vi "Read Payload.vi"(8 "error in (no error)":errorcluster, 11 "RDS Message in":refnum<class "RDS Message.lvclass">) -> (0 "error out":errorcluster, 2 "Payload Out":refnum<class "RDS Payload.lvclass">, 3 "RDS Message out":refnum<class "RDS Message.lvclass">)   [LabVIEW 2015]
uses:
  RDS Message.lvclass
  RDS Payload Class/RDS Payload.lvclass
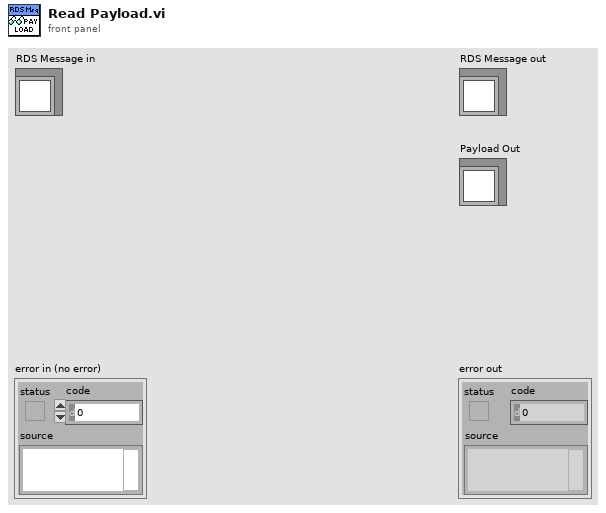
[diagram p1: front panel]
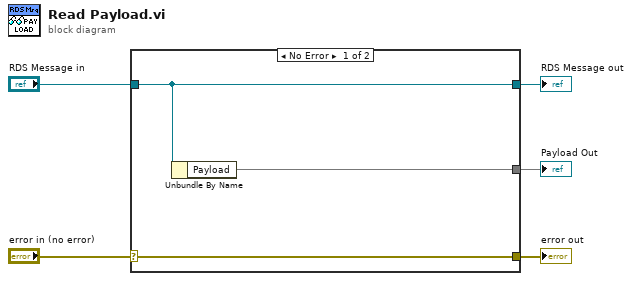
[diagram p0: block diagram]
diagram:
  n1 = case shown="No Error" "error in (no error)" {
    selector: "error in (no error)" -> [w8 w9]
    tunnel: [w8 w9] -> w4
    tunnel: [w7 w10] -> w2
    tunnel: "RDS Message in" -> [w7 w10]
    tunnel: [w6 _] -> w1
    frame No Error {
      n2 = Unbundle By Name(w7) -> ("Payload"=w6)
    }
    frame Error {
    }
  }
  "error out" <- w4
  "RDS Message out" <- w2
  "Payload Out" <- w1
